vi "frequency-test.vi"() -> ()   [LabVIEW 2014]
uses:
  Jiga/stateCtl.ctl
  <vilib>/express/express shared/transition.llb/Dynamic To Waveform Array.vi
  <vilib>/express/express signal manip/GetorSetDDTAttributes/Set DDT Attributes/SetT0.vi
  <vilib>/express/express shared/transition.llb/Waveform Array To Dynamic.vi
  <vilib>/Instr/_visa.llb/VISA Configure Serial Port (Instr).vi
  <vilib>/express/express signal manip/GetorSetDDTAttributes/Set DDT Attributes/Set DDT Properties.xnode
panel:
  out "DT (%)":dbl
  in  "DutyCycleUpperLimit":dbl
  in  "DutyCycleLowerLimit":dbl
  in  "Channel":dbl=1.0 min=1.0 max=2.0 step=1.0
  in  "delay(ms)":dbl=50.0 min=50.0 max=1000.0 step=1.0
  in  "step":dbl
  out "Frequency":dbl(graph)
  out "Analog Output":dbl(graph)
  in  "AnalogOutputDT":dbl(slide) min=31.0 scale=0.0..100.0
  out "S6":dbl
  out "S0":dbl
  out "exitLed":bool
  out "statusBar":string="     "
  in  "startButton":bool
  out "stopLed":bool
  out "startLed":bool
  in  "VISA Serial Port":refnum<visa-resource-name>
  in  "exitButton":bool
  in  "stopButton":bool
  out "FE":string
  out "FP":string
  out "isRunning":bool
  out "state":T1=enum."exit"
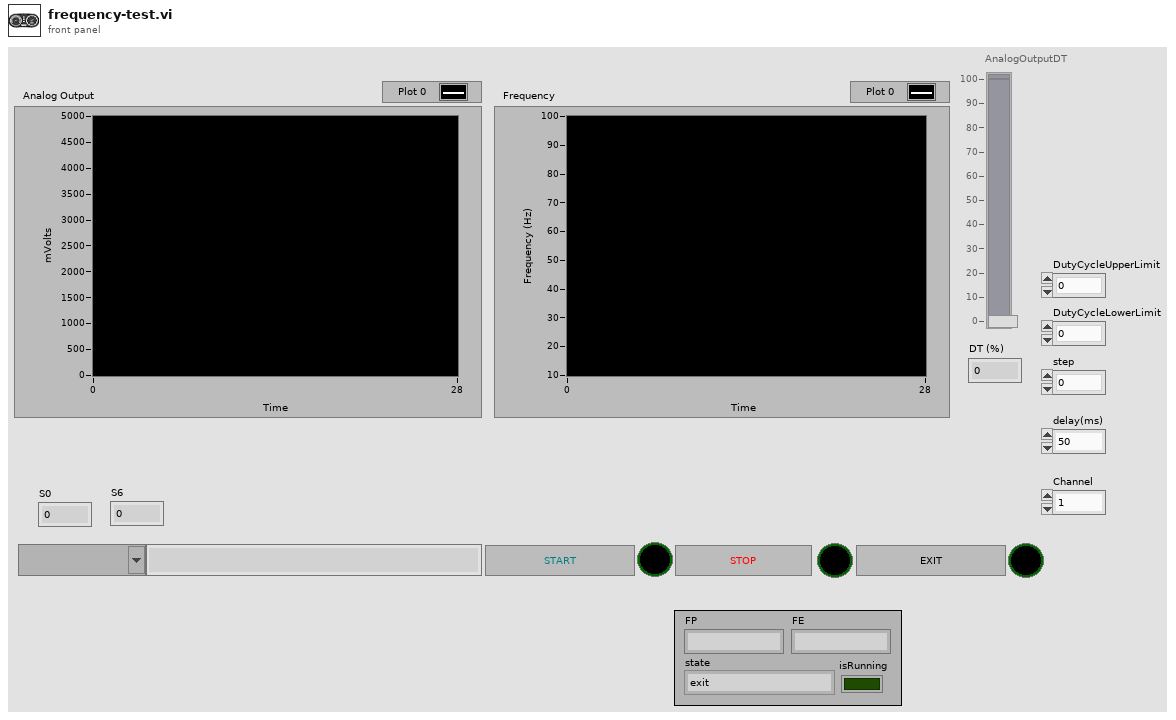
[diagram p1: front panel]
types:
  T1 = typedef "stateCtl.ctl" = enum16{"init", "ready", "running", "stopped", "exit"}
  T2 = enum8{"Enabled", "Disabled", "Disabled and Grayed Out"}
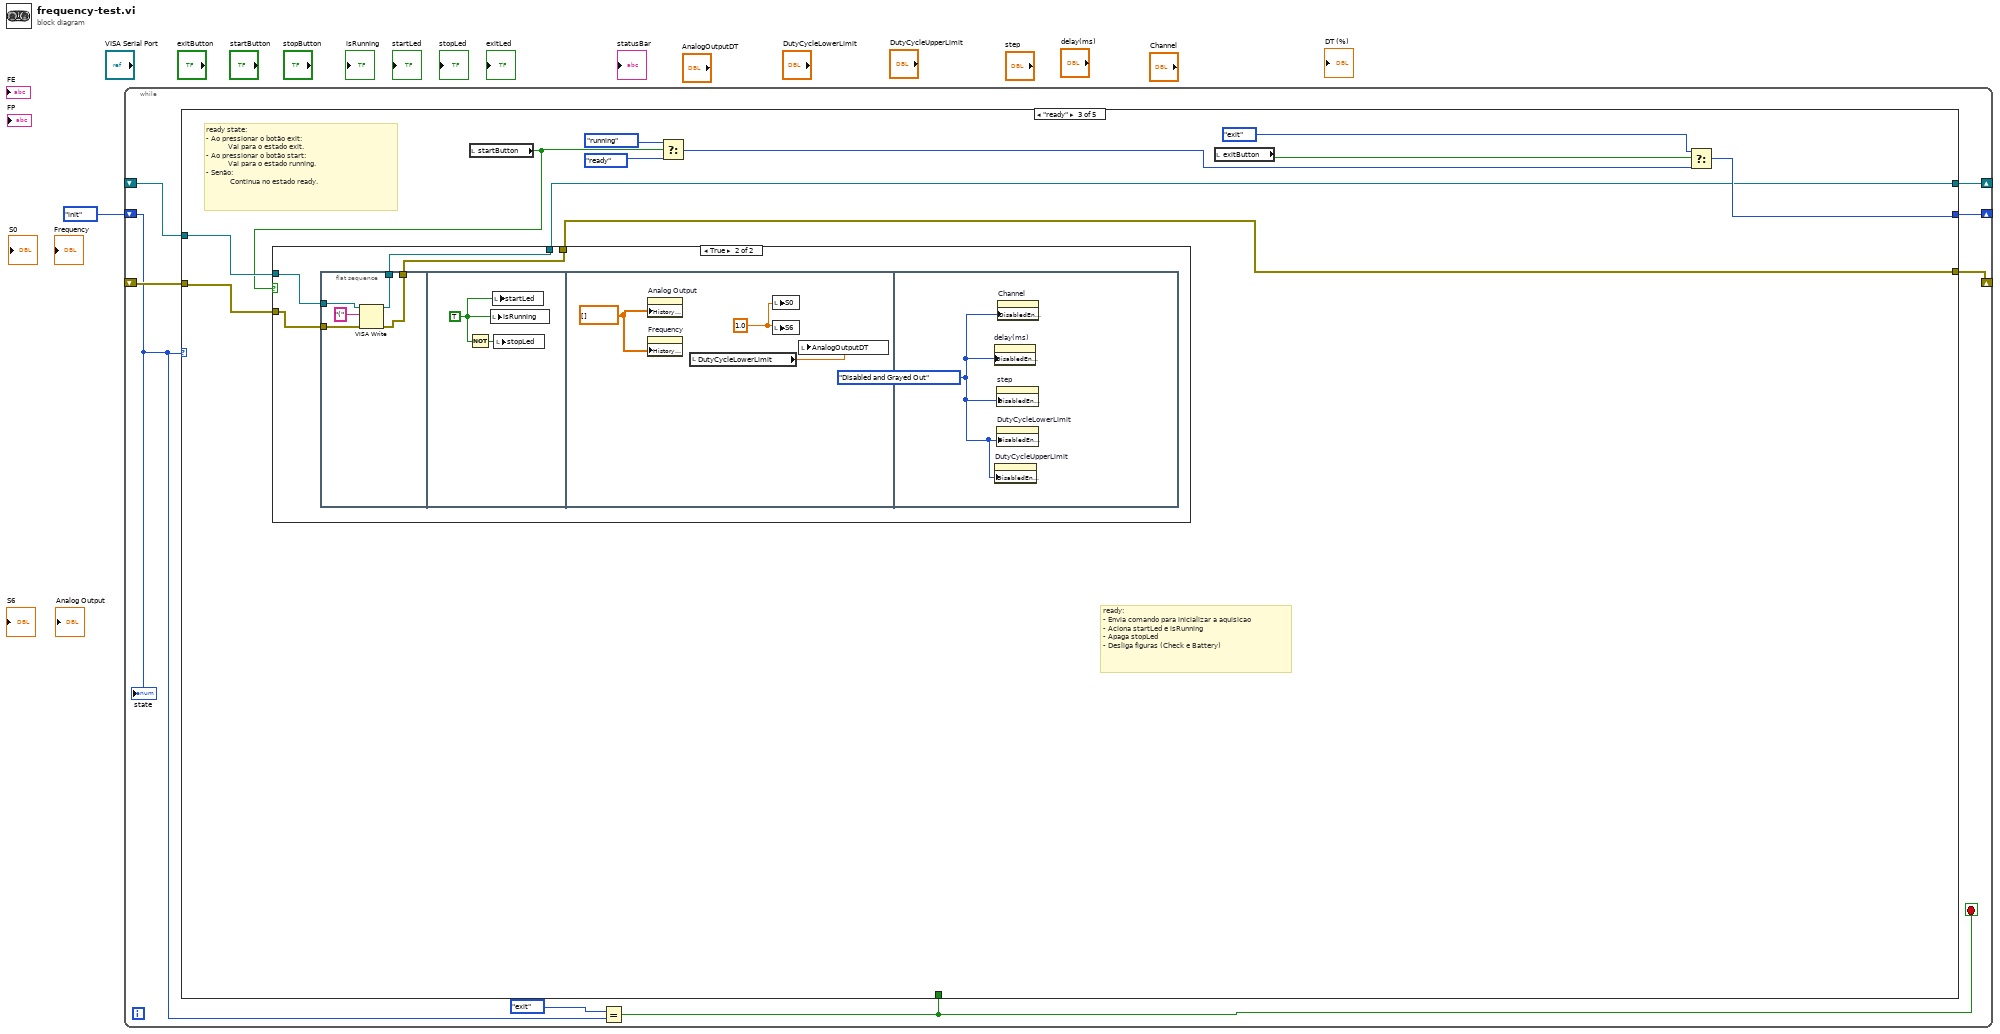
[diagram p0: block diagram]
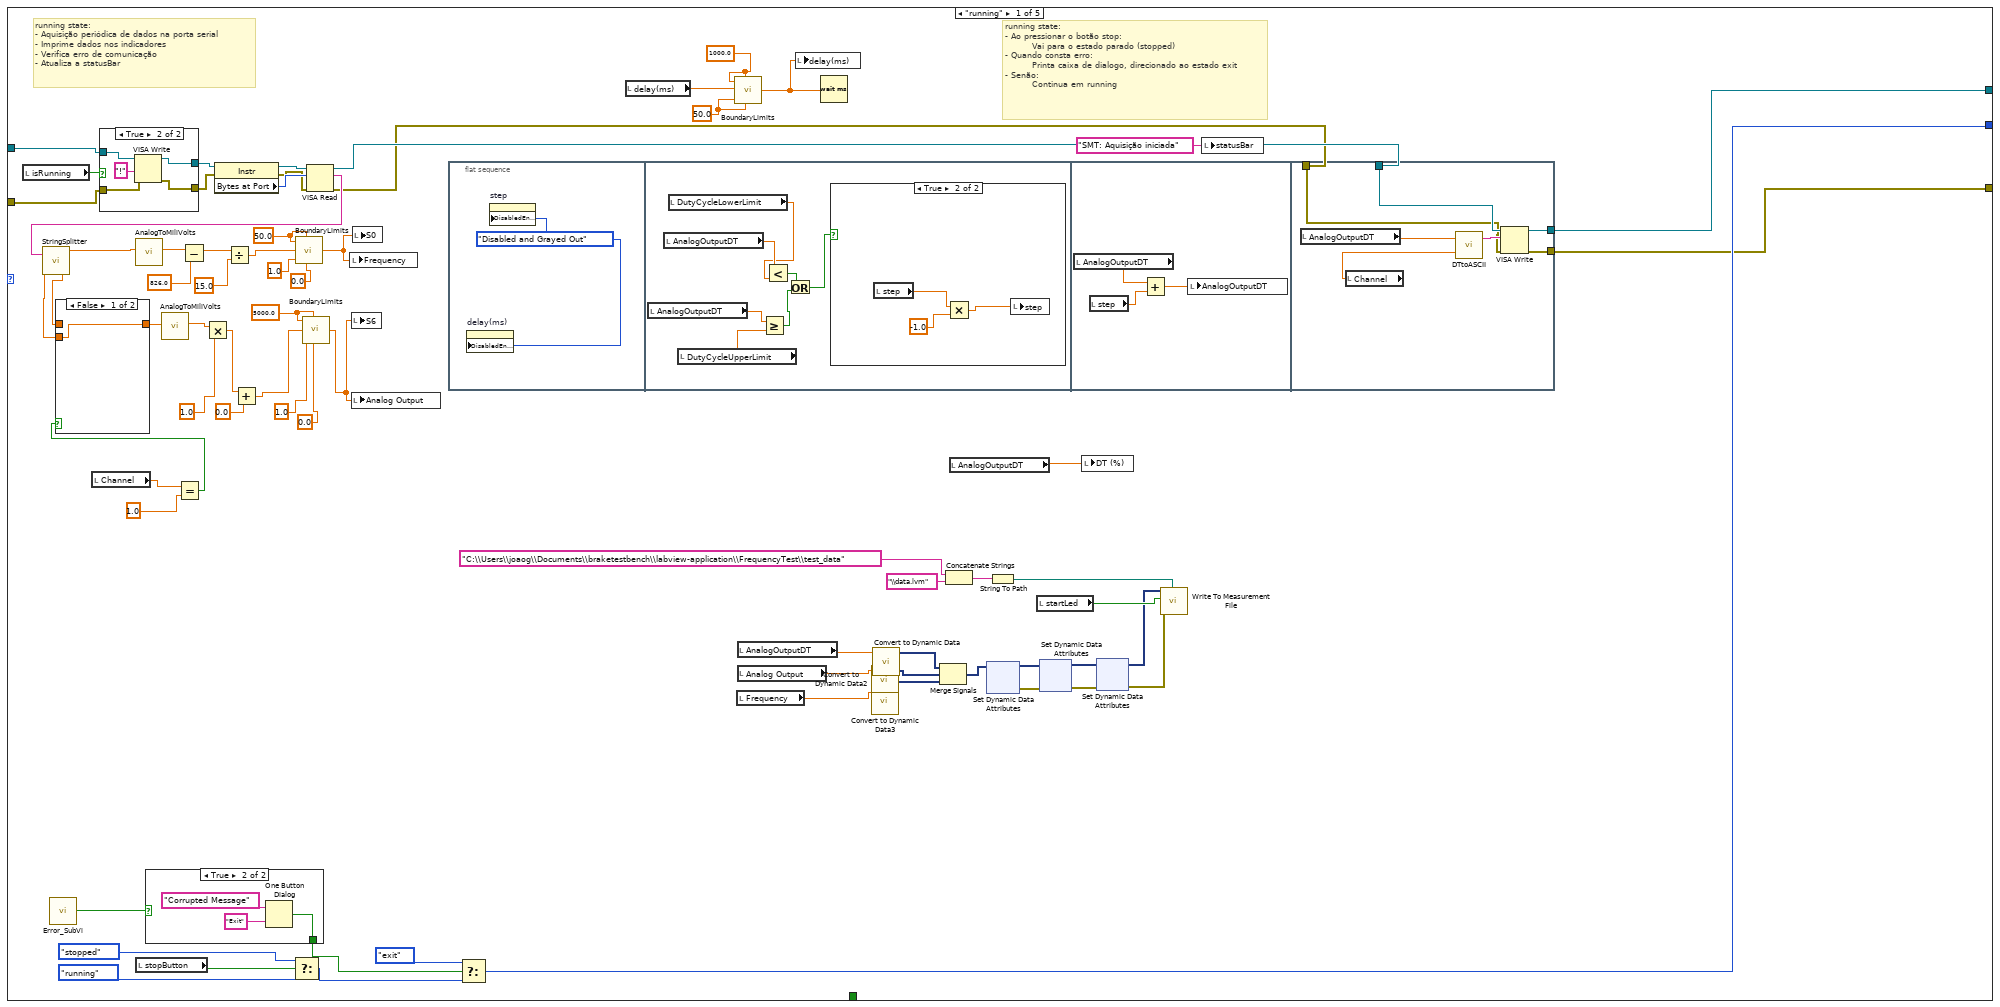
[diagram p2: hidden frame]
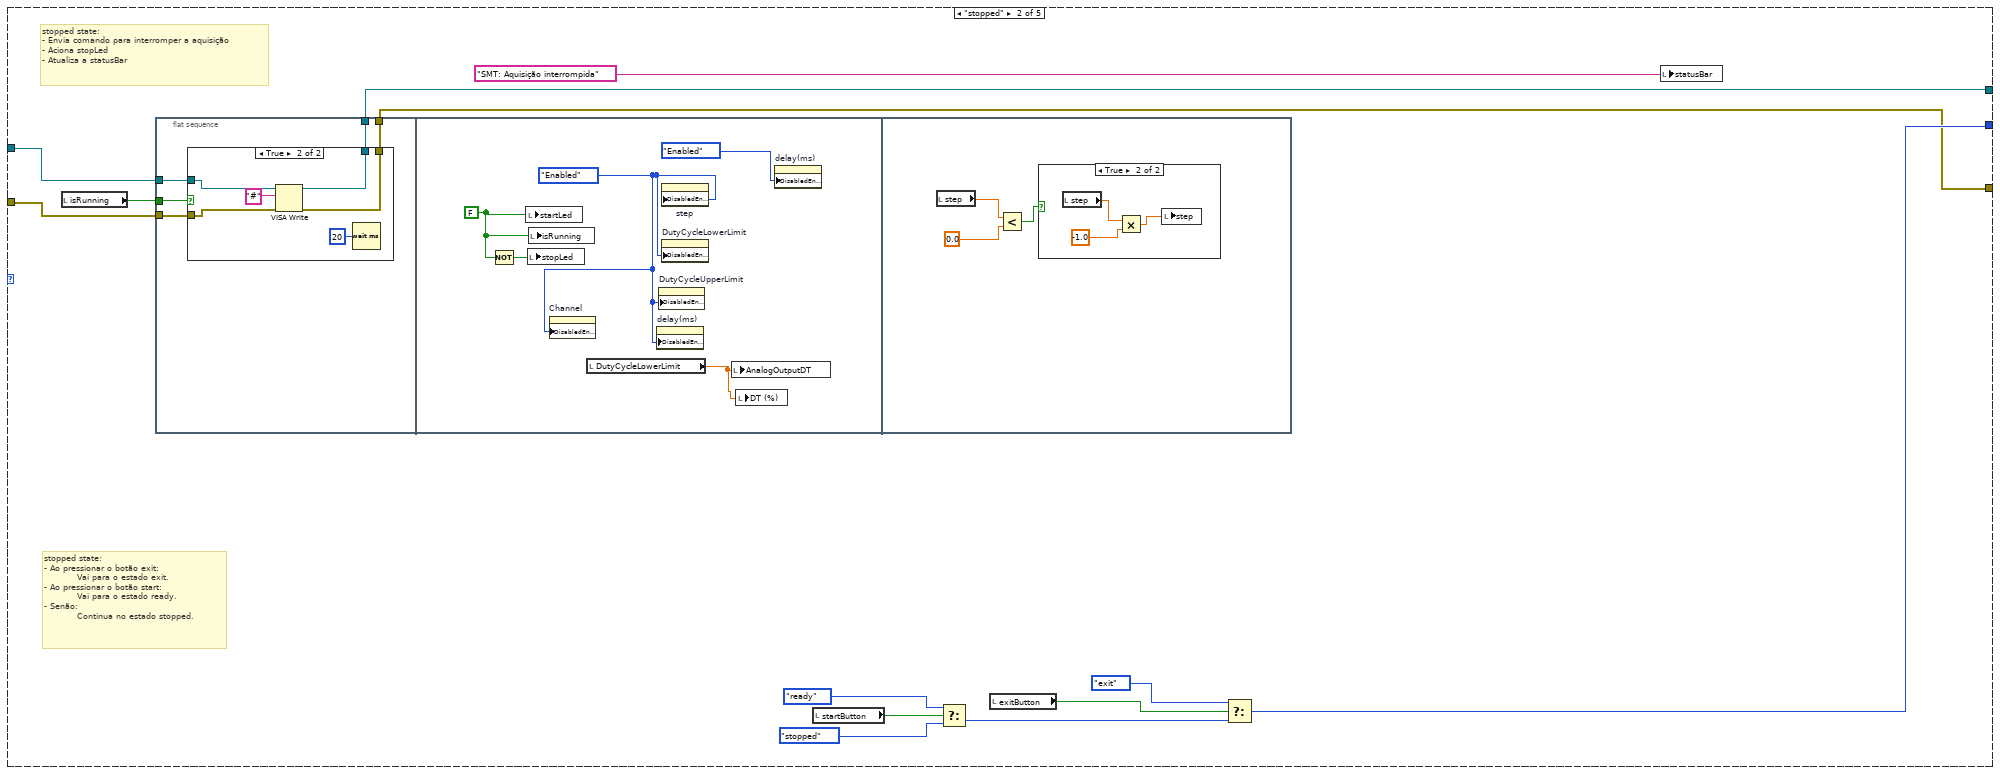
[diagram p7: hidden frame]
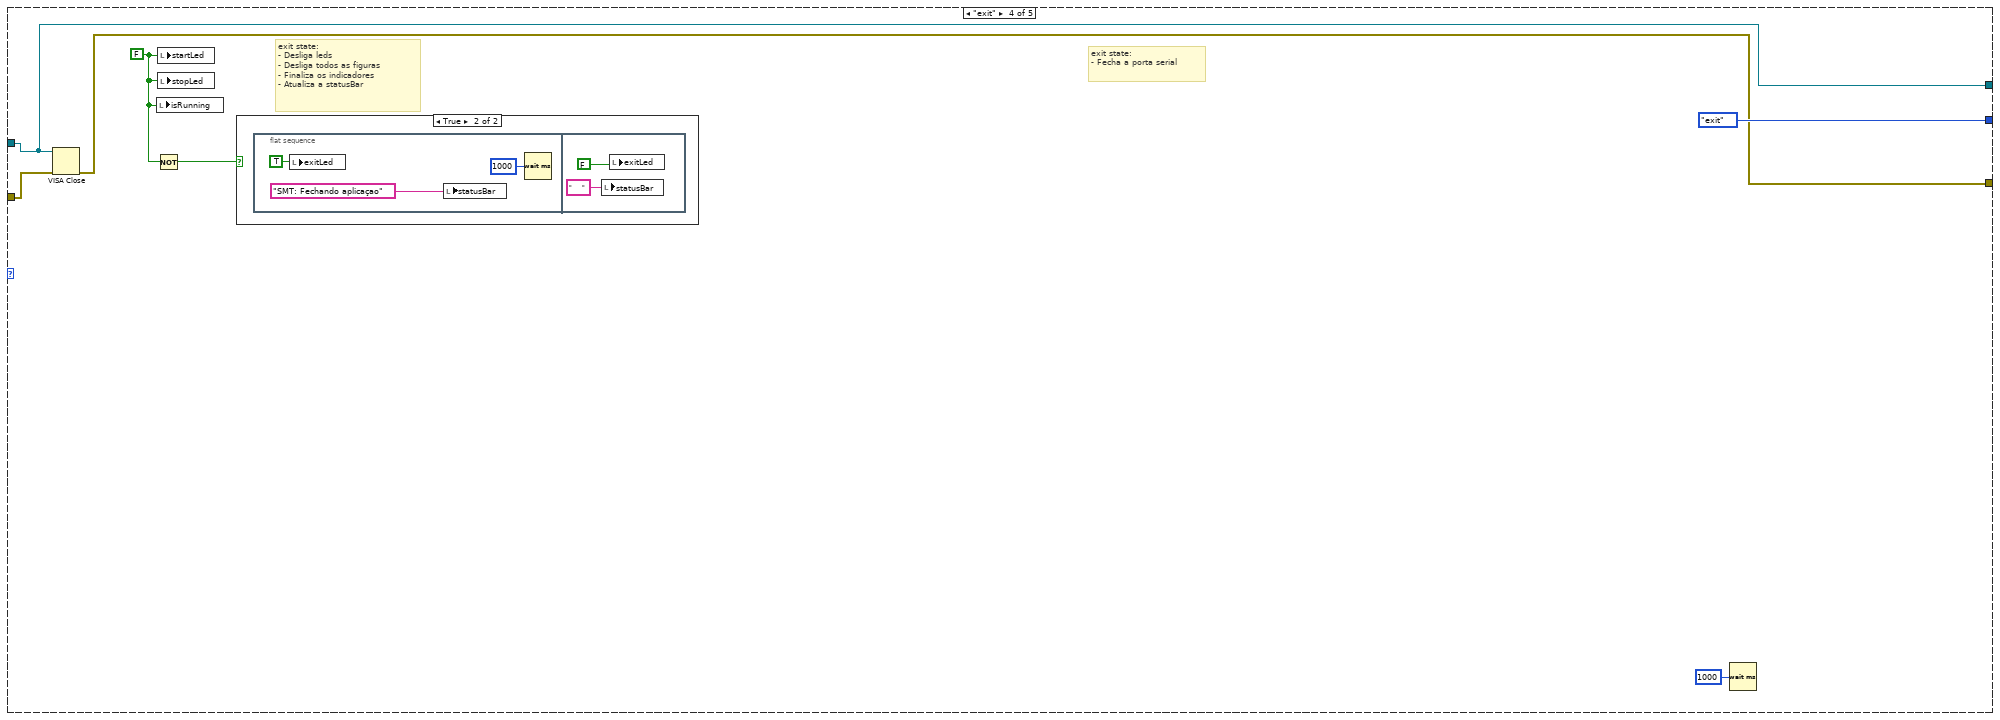
[diagram p11: hidden frame]
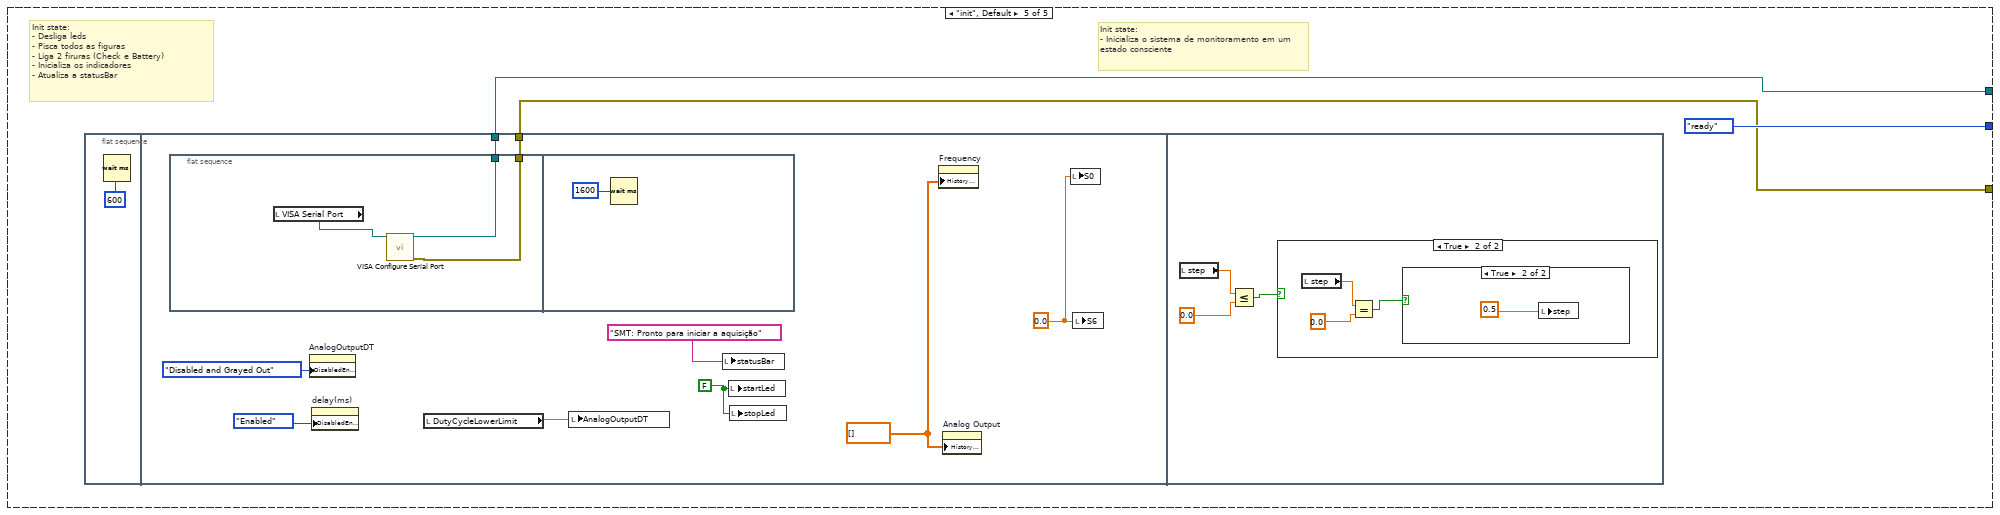
[diagram p13: hidden frame]
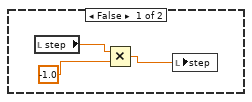
[diagram p15: hidden frame]
diagram:
  n1 = while {
    shift-right: [w3] -> _
    shift-left: _ -> [w8]
    shift-right: [w9] -> _
    shift-left: _ -> [w7]
    shift-right: [w4] -> _
    shift-left: stateCtl."init" ("state") -> [w5]
    stop <- w2 stop-if-true
    n2 = Equal?(x=stateCtl."exit" ("state"), y=w5) -> (x = y?=w2:bool)
    n3 = case shown="\"ready\"" w5 {
      tunnel: [w48 w172 w207 w236 w246] -> w3
      tunnel: [w47 w173 w206 w237 w245] -> w9
      tunnel: [w74 w178 w210 stateCtl."exit" ("state") stateCtl."ready" ("state")] -> w4
      tunnel: w8 -> [w68 w176 w208 w236 _]
      tunnel: w7 -> [w67 w175 w209 w238 _]
      tunnel: w2 -> [_ _ _ _ _]
      frame "running" {
        w12 = 1000.0
        w11 = 50.0
        w57 = 5000.0
        w60 = 50.0
        # "running state:\n- Ao pressionar o botão stop: \n         Vai para o estado parado (stopped)\n- Quando consta erro:\n         Printa caixa de dialogo, direcionado ao estado exit  \n- Senão:          \n         Continua em running"
        # "running state:\n- Aquisição periódica de dados na porta serial\n- Imprime dados nos indicadores\n- Verifica erro de comunicação\n- Atualiza a statusBar"
        n4 = local read "isRunning"() -> (w71:bool)
        n5 = call "Error_SubVi.vi"() -> ("error"=w70:bool)  [unwired: 11 in]
        n6 = local read "Channel"() -> (w39:dbl)
        n7 = case shown="True" w71 {
          tunnel: [w162 w163] -> w65
          tunnel: [w161 w164] -> w66
          tunnel: w67 -> [w162 w166]
          tunnel: w68 -> [w161 w165]
          frame False {
          }
          frame True {
            n8 = VISA Write(VISA resource name=w165, write buffer="!", error in (no error)=w166) -> (VISA resource name out=w164:refnum<visa-resource-name>, error out=w163:errorcluster)  [unwired: 1 out]
          }
        }
        n9 = local read "stopButton"() -> (w78:bool)
        n10 = case shown="True" w70 {
          selector: w70 -> [w157 _]
          tunnel: [w157 w158] -> w72
          frame False {
          }
          frame True {
            n11 = One Button Dialog(message="Corrupted Message", button name ("OK")="Exit") -> (true=w158:bool)
          }
        }
        n12 = Equal?(x=w39, y=1.0) -> (x = y?=w37:bool)
        n13 = property class="Instr"(reference=w66, error in=w65) -> (reference out=w62:refnum<visa-resource-name>, error out=w63:errorcluster, "Bytes at Port"=w64:u32)
        n14 = Select(t=stateCtl."stopped" ("state"), s=w78, f=stateCtl."running" ("state")) -> (s? t:f=w73:T1)
        n15 = VISA Read(VISA resource name=w62, byte count=w64, error in (no error)=w63) -> (VISA resource name out=w50:refnum<visa-resource-name>, read buffer=w61:string, error out=w49:errorcluster)  [unwired: 1 out]
        n16 = call "StringSplitter.vi"("Input String"=w61) -> ("S7"=w41:dbl, "S6"=w42:dbl, "S0"=w35:dbl)  [unwired: 11 in, 5 out]
        n17 = case shown="False" w37 {
          tunnel: w42 -> [_ w135]
          tunnel: w41 -> [w134 _]
          tunnel: [w134 w135] -> w40
          frame False {
          }
          frame True {
          }
        }
        n18 = call "AnalogToMiliVolts.vi"("Input"=w35) -> ("Output"=w34:dbl)  [unwired: 10 in]
        n19 = call "AnalogToMiliVolts.vi"("Input"=w40) -> ("Output"=w43:dbl)  [unwired: 10 in]
        n20 = Subtract(x=w34, y=826.0) -> (x-y=w46:dbl)
        n21 = Multiply(x=w43, y=1.0) -> (x*y=w69:dbl)
        n22 = Divide(x=w46, y=15.0) -> (x/y=w44:dbl)
        n23 = Add(x=w69, y=0.0) -> (x+y=w53:dbl)
        n24 = call "BoundaryLimits.vi"("UpperLimit"=w60, "UpperValue"=w60, "Input"=w44, "LowerLimit"=1.0, "LowerValue"=0.0) -> ("Output"=w36:dbl)
        n25 = call "BoundaryLimits.vi"("UpperLimit"=w57, "UpperValue"=w57, "Input"=w53, "LowerLimit"=1.0, "LowerValue"=0.0) -> ("Output"=w52:dbl)
        n26 = local write "Frequency"(w36) -> ()
        n27 = local write "S6"(w52) -> ()
        n28 = local write "Analog Output"(w52) -> ()
        n29 = local write "S0"(w36) -> ()
        n30 = flat-sequence {
          tunnel: w50 -> [w154]
          tunnel: w49 -> [w153]
          tunnel: [w152] -> w48
          tunnel: [w151] -> w47
          frame #0 {
            w136 = T2."Disabled and Grayed Out" ("Disabled")
            n31 = property on="delay(ms)" class="DigNum (strict)"("DisabledEnum"=w136) -> ()  [unwired: 2 in, 2 out]
            n32 = property on="step" class="DigNum (strict)"("DisabledEnum"=w136) -> ()  [unwired: 2 in, 2 out]
          }
          frame #1 {
            n33 = local read "AnalogOutputDT"() -> (w143:dbl)
            n34 = local read "AnalogOutputDT"() -> (w139:dbl)
            n35 = local read "DutyCycleLowerLimit"() -> (w138:dbl)
            n36 = local read "DutyCycleUpperLimit"() -> (w137:dbl)
            n37 = Greater Or Equal?(x=w143, y=w137) -> (x >= y?=w142:bool)
            n38 = Less?(x=w139, y=w138) -> (x < y?=w140:bool)
            n39 = Or(x=w140, y=w142) -> (x .or. y?=w141:bool)
            n40 = case shown="True" w141 {
              frame False {
              }
              frame True {
                n41 = local read "step"() -> (w145:dbl)
                n42 = Multiply(x=w145, y=-1.0) -> (x*y=w144:dbl)
                n43 = local write "step"(w144) -> ()
              }
            }
          }
          frame #2 {
            n44 = local read "AnalogOutputDT"() -> (w149:dbl)
            n45 = local read "step"() -> (w147:dbl)
            n46 = Add(x=w149, y=w147) -> (x+y=w148:dbl)
            n47 = local write "AnalogOutputDT"(w148) -> ()
          }
          frame #3 {
            n48 = local read "AnalogOutputDT"() -> (w155:dbl)
            n49 = local read "Channel"() -> (w150:dbl)
            n50 = call "DTtoASCII.vi"("Channel"=w150, "Slide"=w155) -> ("ASCII"=w156:string)  [unwired: 1 out]
            n51 = VISA Write(VISA resource name=w154, write buffer=w156, error in (no error)=w153) -> (VISA resource name out=w152:refnum<visa-resource-name>, error out=w151:errorcluster)  [unwired: 1 out]
          }
        }
        n52 = Select(t=stateCtl."exit" ("state"), s=w72, f=w73) -> (s? t:f=w74:T1)
        n53 = local read "delay(ms)"() -> (w13:dbl)
        n54 = call "BoundaryLimits.vi"("UpperLimit"=w12, "UpperValue"=w12, "Input"=w13, "LowerLimit"=w11, "LowerValue"=w11) -> ("Output"=w10:dbl)
        n55 = local read "Frequency"() -> (w27:dbl)
        n56 = local read "AnalogOutputDT"() -> (w16:dbl)
        n57 = local read "Analog Output"() -> (w26:dbl)
        n58 = local write "delay(ms)"(w10) -> ()
        n59 = Wait (ms)(milliseconds to wait=w10) -> ()  [unwired: 1 out]
        n60 = call "Convert to Dynamic Data2"("Double"=w26) -> ("Dynamic Data Type"=w24:dynamicdata)  [unwired: 3 in]
        n61 = call "Convert to Dynamic Data3"("Double"=w27) -> ("Dynamic Data Type"=w25:dynamicdata)  [unwired: 3 in]
        n62 = call "Convert to Dynamic Data"("Double"=w16) -> ("Dynamic Data Type"=w23:dynamicdata)  [unwired: 3 in]
        n63 = Merge Signals(w23, w24, w25) -> (w19:dynamicdata)
        n64 = Concatenate Strings("C:\\Users\\joaog\\Documents\\braketestbench\\labview-application\\FrequencyTest\\test_data", "\\data.lvm" ("string")) -> (w28:string)
        n65 = local read "AnalogOutputDT"() -> (w15:dbl)
        n66 = xnode ("Set Dynamic Data Attributes")("Signals In"=w19) -> ("Signals Out"=w14:dynamicdata, "error out"=w20:errorcluster)  [unwired: 4 in]
        n67 = String To Path(string=w28) -> (path=w30:path)
        n68 = local read "startLed"() -> (w32:bool)
        n69 = xnode ("Set Dynamic Data Attributes")("Signals In"=w14, "error in"=w20) -> ("Signals Out"=w18:dynamicdata, "error out"=w21:errorcluster)  [unwired: 3 in]
        n70 = local write "DT (%)"(w15) -> ()
        n71 = xnode ("Set Dynamic Data Attributes")("Signals In"=w18, "error in"=w21) -> ("Signals Out"=w17:dynamicdata, "error out"=w22:errorcluster)  [unwired: 3 in]
        n72 = call "Write To Measurement File"("Signals"=w17, "Enable"=w32, "error in (no error)"=w22, "Filename"=w30) -> ()  [unwired: 13 in, 3 out]
        n73 = local write "statusBar"("SMT: Aquisição iniciada" ("statusBar")) -> ()
      }
      frame "stopped" {
        # "stopped state:\n- Ao pressionar o botão exit: \n           Vai para o estado exit.\n- Ao pressionar o botão start:\n           Vai para o estado ready.\n- Senão:\n           Continua no estado stopped."
        # "stopped state:\n- Envia comando para interromper a aquisição\n- Aciona stopLed\n- Atualiza a statusBar"
        n74 = local read "isRunning"() -> (w174:bool)
        n75 = flat-sequence {
          tunnel: w176 -> [w185]
          tunnel: w175 -> [w184]
          tunnel: w174 -> [w183]
          tunnel: [w182] -> w173
          tunnel: [w181] -> w172
          frame #0 {
            n76 = case shown="True" w183 {
              tunnel: w185 -> [w187 w193]
              tunnel: w184 -> [w186 w192]
              tunnel: [w186 w188] -> w182
              tunnel: [w187 w190] -> w181
              frame False {
              }
              frame True {
                n77 = VISA Write(VISA resource name=w193, write buffer="#", error in (no error)=w192) -> (VISA resource name out=w190:refnum<visa-resource-name>, error out=w188:errorcluster)  [unwired: 1 out]
                n78 = Wait (ms)(milliseconds to wait=u32 20) -> ()  [unwired: 1 out]
              }
            }
          }
          frame #1 {
            w194 = T2."Enabled" ("Disabled")
            w197 = FALSE ("Boolean")
            n79 = Not(x=w197) -> (.not. x?=w198:bool)
            n80 = local write "startLed"(w197) -> ()
            n81 = local write "stopLed"(w198) -> ()
            n82 = local write "isRunning"(w197) -> ()
            n83 = property on="Channel" class="DigNum (strict)"("DisabledEnum"=w194) -> ()  [unwired: 2 in, 2 out]
            n84 = local read "DutyCycleLowerLimit"() -> (w195:dbl)
            n85 = property on="delay(ms)" class="DigNum (strict)"("DisabledEnum"=w194) -> ()  [unwired: 2 in, 2 out]
            n86 = property on="DutyCycleUpperLimit" class="DigNum (strict)"("DisabledEnum"=w194) -> ()  [unwired: 2 in, 2 out]
            n87 = property on="step" class="DigNum (strict)"("DisabledEnum"=w194) -> ()  [unwired: 2 in, 2 out]
            n88 = property on="DutyCycleLowerLimit" class="DigNum (strict)"("DisabledEnum"=w194) -> ()  [unwired: 2 in, 2 out]
            n89 = local write "AnalogOutputDT"(w195) -> ()
            n90 = local write "DT (%)"(w195) -> ()
            n91 = property on="delay(ms)" class="DigNum (strict)"("DisabledEnum"=T2."Enabled" ("Disabled")) -> ()  [unwired: 2 in, 2 out]
          }
          frame #2 {
            n92 = local read "step"() -> (w200:dbl)
            n93 = Less?(x=w200, y=0.0) -> (x < y?=w199:bool)
            n94 = case shown="True" w199 {
              frame False {
              }
              frame True {
                n95 = local read "step"() -> (w204:dbl)
                n96 = Multiply(x=w204, y=-1.0) -> (x*y=w202:dbl)
                n97 = local write "step"(w202) -> ()
              }
            }
          }
        }
        n98 = local read "startButton"() -> (w171:bool)
        n99 = Select(t=stateCtl."ready" ("state"), s=w171, f=stateCtl."stopped" ("state")) -> (s? t:f=w179:T1)
        n100 = local read "exitButton"() -> (w170:bool)
        n101 = Select(t=stateCtl."exit" ("state"), s=w170, f=w179) -> (s? t:f=w178:T1)
        n102 = local write "statusBar"("SMT: Aquisição interrompida" ("statusBar")) -> ()
      }
      frame "ready" {
        # "ready state:\n- Ao pressionar o botão exit: \n           Vai para o estado exit.\n- Ao pressionar o botão start:\n           Vai para o estado running.\n- Senão:\n            Continua no estado ready."
        # "ready:\n- Envia comando para inicializar a aquisicao\n- Aciona startLed e isRunning\n- Apaga stopLed\n- Desliga figuras (Check e Battery)"
        n103 = local read "startButton"() -> (w205:bool)
        n104 = case shown="True" w205 {
          tunnel: [w217 w221] -> w207
          tunnel: [w216 w220] -> w206
          tunnel: w208 -> [w217 w219]
          tunnel: w209 -> [w216 w218]
          frame False {
          }
          frame True {
            n105 = flat-sequence {
              tunnel: [w225] -> w221
              tunnel: [w224] -> w220
              tunnel: w219 -> [w223]
              tunnel: w218 -> [w222]
              frame #0 {
                n106 = VISA Write(VISA resource name=w223, write buffer="(", error in (no error)=w222) -> (VISA resource name out=w225:refnum<visa-resource-name>, error out=w224:errorcluster)  [unwired: 1 out]
              }
              frame #1 {
                w228 = TRUE ("Boolean")
                n107 = Not(x=w228) -> (.not. x?=w227:bool)
                n108 = local write "isRunning"(w228) -> ()
                n109 = local write "startLed"(w228) -> ()
                n110 = local write "stopLed"(w227) -> ()
              }
              frame #2 {
                w230 = 1.0
                w231 = dbl[] [] ("History Data")
                n111 = property on="Analog Output" class="WFChart (strict)"("History Data"=w231) -> ()  [unwired: 2 in, 2 out]
                n112 = property on="Frequency" class="WFChart (strict)"("History Data"=w231) -> ()  [unwired: 2 in, 2 out]
                n113 = local read "DutyCycleLowerLimit"() -> (w229:dbl)
                n114 = local write "S0"(w230) -> ()
                n115 = local write "S6"(w230) -> ()
                n116 = local write "AnalogOutputDT"(w229) -> ()
              }
              frame #3 {
                w232 = T2."Disabled and Grayed Out" ("Disabled")
                n117 = property on="delay(ms)" class="DigNum (strict)"("DisabledEnum"=w232) -> ()  [unwired: 2 in, 2 out]
                n118 = property on="DutyCycleUpperLimit" class="DigNum (strict)"("DisabledEnum"=w232) -> ()  [unwired: 2 in, 2 out]
                n119 = property on="step" class="DigNum (strict)"("DisabledEnum"=w232) -> ()  [unwired: 2 in, 2 out]
                n120 = property on="DutyCycleLowerLimit" class="DigNum (strict)"("DisabledEnum"=w232) -> ()  [unwired: 2 in, 2 out]
                n121 = property on="Channel" class="DigNum (strict)"("DisabledEnum"=w232) -> ()  [unwired: 2 in, 2 out]
              }
            }
          }
        }
        n122 = Select(t=stateCtl."running" ("state"), s=w205, f=stateCtl."ready" ("state")) -> (s? t:f=w211:T1)
        n123 = local read "exitButton"() -> (w213:bool)
        n124 = Select(t=stateCtl."exit" ("state"), s=w213, f=w211) -> (s? t:f=w210:T1)
      }
      frame "exit" {
        w234 = FALSE ("startLed")
        # "exit state:\n- Desliga leds\n- Desliga todos as figuras\n- Finaliza os indicadores\n- Atualiza a statusBar"
        # "exit state:\n- Fecha a porta serial"
        n125 = VISA Close(VISA resource name=w236, error in (no error)=w238) -> (error out=w237:errorcluster)
        n126 = Not(x=w234) -> (.not. x?=w235:bool)
        n127 = local write "isRunning"(w234) -> ()
        n128 = local write "startLed"(w234) -> ()
        n129 = local write "stopLed"(w234) -> ()
        n130 = case shown="True" w235 {
          frame False {
          }
          frame True {
            n131 = flat-sequence {
              frame #0 {
                n132 = local write "exitLed"(TRUE ("exitLed")) -> ()
                n133 = local write "statusBar"("SMT: Fechando aplicaçao" ("statusBar")) -> ()
                n134 = Wait (ms)(milliseconds to wait=u32 1000) -> ()  [unwired: 1 out]
              }
              frame #1 {
                n135 = local write "statusBar"("     " ("statusBar")) -> ()
                n136 = local write "exitLed"(FALSE ("exitLed")) -> ()
              }
            }
          }
        }
        n137 = Wait (ms)(milliseconds to wait=u32 1000) -> ()  [unwired: 1 out]
      }
      frame "init", Default {
        # "Init state:\n- Inicializa o sistema de monitoramento em um estado consciente"
        # "Init state:\n- Desliga leds\n- Pisca todos as figuras\n- Liga 2 firuras (Check e Battery)\n- Inicializa os indicadores\n- Atualiza a statusBar"
        n138 = flat-sequence {
          tunnel: [w252] -> w246
          tunnel: [w251] -> w245
          frame #0 {
            n139 = Wait (ms)(milliseconds to wait=u32 600) -> ()  [unwired: 1 out]
          }
          frame #1 {
            w255 = dbl[] [] ("History Data")
            w254 = 0.0
            w257 = FALSE
            n140 = flat-sequence {
              tunnel: [w259] -> w252
              tunnel: [w258] -> w251
              frame #0 {
                n141 = local read "VISA Serial Port"() -> (w260:refnum<visa-resource-name>)
                n142 = call-poly "VISA Configure Serial Port"("VISA resource name"=w260) -> ("VISA resource name out"=w259:refnum<visa-resource-name>, "error out"=w258:errorcluster)  [unwired: 13 in]
              }
              frame #1 {
                n143 = Wait (ms)(milliseconds to wait=u32 1600) -> ()  [unwired: 1 out]
              }
            }
            n144 = property on="AnalogOutputDT" class="Slide (strict)"("DisabledEnum"=T2."Disabled and Grayed Out" ("Disabled")) -> ()  [unwired: 2 in, 2 out]
            n145 = property on="delay(ms)" class="DigNum (strict)"("DisabledEnum"=T2."Enabled" ("Disabled")) -> ()  [unwired: 2 in, 2 out]
            n146 = local read "DutyCycleLowerLimit"() -> (w250:dbl)
            n147 = local write "AnalogOutputDT"(w250) -> ()
            n148 = local write "statusBar"("SMT: Pronto para iniciar a aquisição" ("statusBar")) -> ()
            n149 = local write "startLed"(w257) -> ()
            n150 = local write "stopLed"(w257) -> ()
            n151 = property on="Frequency" class="WFChart (strict)"("History Data"=w255) -> ()  [unwired: 2 in, 2 out]
            n152 = property on="Analog Output" class="WFChart (strict)"("History Data"=w255) -> ()  [unwired: 2 in, 2 out]
            n153 = local write "S0"(w254) -> ()
            n154 = local write "S6"(w254) -> ()
          }
          frame #2 {
            n155 = local read "step"() -> (w264:dbl)
            n156 = Less Or Equal?(x=w264, y=0.0) -> (x <= y?=w262:bool)
            n157 = case shown="True" w262 {
              frame False {
              }
              frame True {
                n158 = local read "step"() -> (w267:dbl)
                n159 = Equal?(x=w267, y=0.0) -> (x = y?=w265:bool)
                n160 = case shown="True" w265 {
                  frame False {
                    n161 = local read "step"() -> (w270:dbl)
                    n162 = Multiply(x=w270, y=-1.0) -> (x*y=w268:dbl)
                    n163 = local write "step"(w268) -> ()
                  }
                  frame True {
                    n164 = local write "step"(0.5) -> ()
                  }
                }
              }
            }
          }
        }
      }
    }
    "state" <- w5
  }
